vi "log_motor_moves.vi"(6 "semaphore":T1, 7 "waypoint version":bool, 8 "error in (no error)":errorcluster, 10 "Answer":string, 11 "VISA resource name":refnum<visa-resource-name>) -> (0 "error out":errorcluster, 2 "Log File":string, 3 "VISA resource name out":refnum<visa-resource-name>)   [LabVIEW 2013]
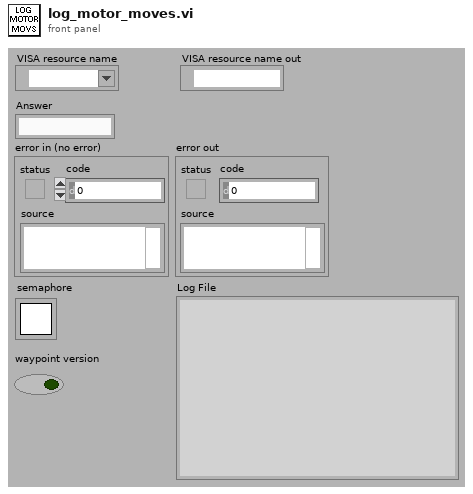
[diagram p1: front panel]
types:
  T1 = typedef "Semaphore RefNum" = refnum<k1>
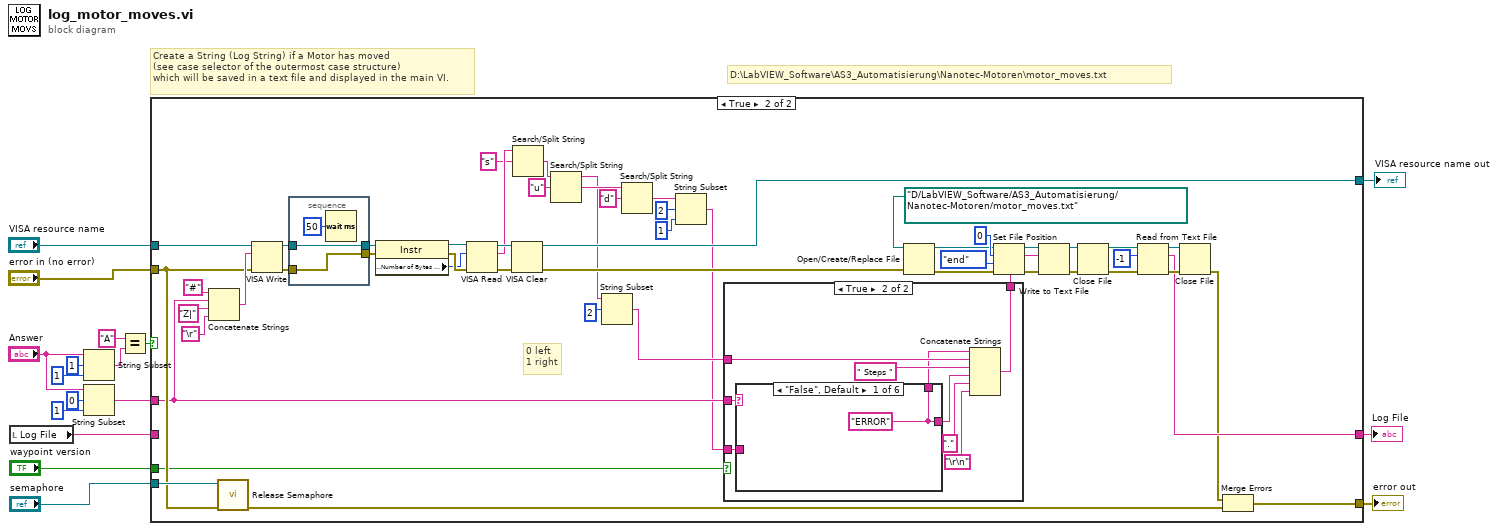
[diagram p0: block diagram]
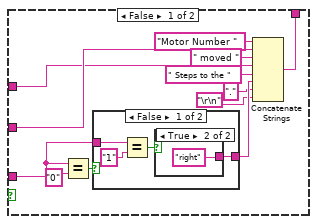
[diagram p3: hidden frame]
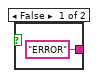
[diagram p4: hidden frame]
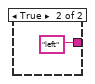
[diagram p5: hidden frame]
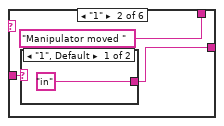
[diagram p6: hidden frame]
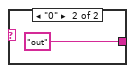
[diagram p7: hidden frame]
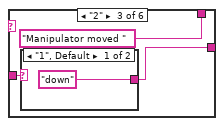
[diagram p8: hidden frame]
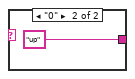
[diagram p9: hidden frame]
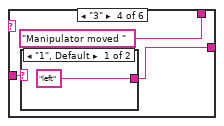
[diagram p10: hidden frame]
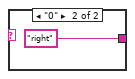
[diagram p11: hidden frame]
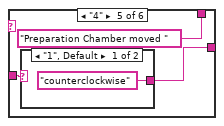
[diagram p12: hidden frame]
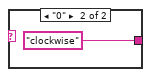
[diagram p13: hidden frame]
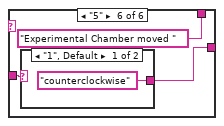
[diagram p14: hidden frame]
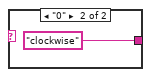
[diagram p15: hidden frame]
diagram:
  # "D:\\LabVIEW_Software\\AS3_Automatisierung\\Nanotec-Motoren\\motor_moves.txt"
  # "Create a String (Log String) if a Motor has moved\n(see case selector of the outermost case structure)\nwhich will be saved in a text file and displayed in the main VI."
  n1 = local read "Log File"() -> (w5:string)
  n2 = String Subset(string="Answer", offset (0)=1, length (rest)=1 ("length (rest)")) -> (substring=w14:string)
  n3 = String Subset(string="Answer", offset (0)=0, length (rest)=1 ("length (rest)")) -> (substring=w7:string)
  n4 = Equal?(x="A", y=w14) -> (x = y?=w13:bool)
  n5 = case shown="True" w13 {
    tunnel: "VISA resource name" -> [w20 w61]
    tunnel: "error in (no error)" -> [w18 w36]
    tunnel: w7 -> [_ w30]
    tunnel: [w20 w40] -> w6
    tunnel: w5 -> [w19 _]
    tunnel: [w19 w38] -> w4
    tunnel: "semaphore" -> [_ w37]
    tunnel: [w18 w33] -> w2
    tunnel: "waypoint version" -> [_ w25]
    frame False {
    }
    frame True {
      # "0 left\n1 right"
      n6 = Concatenate Strings("#" ("staticText"), w30, "Z|" ("Command"), "\r") -> (w62:string)
      n7 = call <vilib>:"Release Semaphore.vi"("error in (no error)"=w36, "semaphore"=w37) -> ("error out"=w35:errorcluster)  [unwired: 4 in, 1 out]
      n8 = VISA Write(VISA resource name=w61, write buffer=w62, error in (no error)=w36) -> (VISA resource name out=w66:refnum<visa-resource-name>, error out=w64:errorcluster)  [unwired: 1 out]
      n9 = stacked-sequence {
        tunnel: w66 -> [w129]
        tunnel: [w129] -> w65
        tunnel: w64 -> [w128]
        tunnel: [w128] -> w63
        frame #0 {
          n10 = Wait (ms)(milliseconds to wait=u32 50) -> ()  [unwired: 1 out]
        }
      }
      n11 = property class="Instr"(reference=w65, error in=w63) -> (reference out=w68:refnum<visa-resource-name>, error out=w69:errorcluster, "Serial Settings:Number of Bytes at Serial Port"=w67:u32)
      n12 = VISA Read(VISA resource name=w68, byte count=w67, error in (no error)=w69) -> (VISA resource name out=w71:refnum<visa-resource-name>, read buffer=w60:string, error out=w70:errorcluster)  [unwired: 1 out]
      n13 = VISA Clear(VISA resource name=w71, error in (no error)=w70) -> (VISA resource name out=w40:refnum<visa-resource-name>, error out=w39:errorcluster)
      n14 = Search/Split String(string=w60, search string/char (-)="s") -> (match + rest of string=w56:string)  [unwired: 1 in, 2 out]
      n15 = Search/Split String(string=w56, search string/char (-)="u") -> (substring before match=w29:string, match + rest of string=w55:string)  [unwired: 1 in, 1 out]
      n16 = String Subset(string=w29, offset (0)=2) -> (substring=w28:string)  [unwired: 1 in]
      n17 = Search/Split String(string=w55, search string/char (-)="d") -> (match + rest of string=w24:string)  [unwired: 1 in, 2 out]
      n18 = String Subset(string=w24, offset (0)=2 ("Offset (0)"), length (rest)=1 ("Länge (Rest)")) -> (substring=w21:string)
      n19 = case shown="True" w25 {
        tunnel: w21 -> [w74 w93]
        tunnel: [w78 w100] -> w41
        tunnel: w30 -> [w77 w95]
        tunnel: w28 -> [w73 w99]
        frame False {
          n20 = Equal?(x=w74, y="0") -> (x = y?=w80:bool)
          n21 = case shown="False" w80 {
            tunnel: w74 -> [w88 _]
            tunnel: [w85 "left" ("y")] -> w79
            frame False {
              n22 = Equal?(x=w88, y="1") -> (x = y?=w86:bool)
              n23 = case shown="True" w86 {
                tunnel: ["ERROR" ("y") "right" ("y")] -> w85
                frame False {
                }
                frame True {
                }
              }
            }
            frame True {
            }
          }
          n24 = Concatenate Strings("Motor Number " ("string"), w77, " moved " ("string"), w73, " Steps to the " ("string"), w79, "." ("string"), "\r\n") -> (w78:string)
        }
        frame True {
          n25 = case shown="\"False\", Default" w95 {
            tunnel: [w101 "Manipulator moved " ("string") "Manipulator moved " ("string") "Manipulator moved " ("string") "Preparation Chamber moved " "Experimental Chamber moved "] -> w94
            tunnel: [w101 w102 w107 w112 w117 w122] -> w92
            tunnel: w93 -> [_ w103 w108 w113 w118 w123]
            frame "False", Default {
              w101 = "ERROR"
            }
            frame "1" {
              n26 = case shown="\"1\", Default" w103 {
                tunnel: ["in" "out"] -> w102
                frame "1", Default {
                }
                frame "0" {
                }
              }
            }
            frame "2" {
              n27 = case shown="\"1\", Default" w108 {
                tunnel: ["down" "up"] -> w107
                frame "1", Default {
                }
                frame "0" {
                }
              }
            }
            frame "3" {
              n28 = case shown="\"1\", Default" w113 {
                tunnel: ["left" "right"] -> w112
                frame "1", Default {
                }
                frame "0" {
                }
              }
            }
            frame "4" {
              n29 = case shown="\"1\", Default" w118 {
                tunnel: ["counterclockwise" "clockwise"] -> w117
                frame "1", Default {
                }
                frame "0" {
                }
              }
            }
            frame "5" {
              n30 = case shown="\"1\", Default" w123 {
                tunnel: ["counterclockwise" "clockwise"] -> w122
                frame "1", Default {
                }
                frame "0" {
                }
              }
            }
          }
          n31 = Concatenate Strings(w94, w99, " Steps " ("string"), w92, "." ("string"), "\r\n") -> (w100:string)
        }
      }
      n32 = Open/Create/Replace File(file path (use dialog)=path "D:/LabVIEW_Software/AS3_Automatisierung/Nanotec-Motoren/motor_moves.txt", error in=w39) -> (refnum out=w49:refnum<file>, error out=w50:errorcluster)  [unwired: 4 in, 1 out]
      n33 = Set File Position(offset (in bytes) (0)=i64 0, refnum=w49, from (0:start)=enum16{"start", "end", "current"}."end", error in=w50) -> (refnum out=w51:refnum<file>, error out=w52:errorcluster)
      n34 = Write to Text File(file (use dialog)=w51, text=w41, error in=w52) -> (refnum out=w45:refnum<file>, error out=w46:errorcluster)  [unwired: 1 in, 1 out]
      n35 = Close File(refnum=w45, error in=w46) -> (path=w47:path, error out=w48:errorcluster)
      n36 = Read from Text File(file (use dialog)=w47, count=-1, error in=w48) -> (refnum out=w42:refnum<file>, text=w38:string, error out=w43:errorcluster)  [unwired: 1 in, 1 out]
      n37 = Close File(refnum=w42, error in=w43) -> (error out=w34:errorcluster)  [unwired: 1 out]
      n38 = Merge Errors(w34, w35) -> (w33:errorcluster)
    }
  }
  "VISA resource name out" <- w6
  "error out" <- w2
  "Log File" <- w4
